vi "校准设置页.vi"() -> ()   [LabVIEW 2016, in "斯坦道氨氮.lvlib"]
uses:
  <vilib>/Analysis/6fits.llb/Curve Fitting Criteria.ctl
  <vilib>/Analysis/NI_AALPro.lvlib
  <vilib>/ptbypt/NI_PtbyPt.lvlib
panel:
  in  "历史数据导入":T1(radio)
  out "校准状态显示":string caption="校准状态"
  out "刷新时间":string
  out "校准状态":T2(ring)
  out "模型刷新":bool
  in  "校准按钮":T1(radio)
  in  "校准导入":bool
  in  "辅助计算":bool
  in  "曲线模型":T3={"标液浓度1"=0.0, "测量吸光度1"=0.0, "样品1启用"=FALSE, "标液浓度2"=0.0, "测量吸光度2"=0.0, "样品2启用"=FALSE, "标液浓度3"=0.0, "测量吸光度3"=0.0, "样品3启用"=FALSE, "标液浓度4"=0.0, "测量吸光度4"=0.0, "样品4启用"=FALSE, "标液浓度5"=0.0, "测量吸光度5"=0.0, "样品5启用"=FALSE, "模型"=enum."线性", "精度"=4.0, "XY图"=[], "拟合公式"="", "r^2"=0.0, "标样一校准时间"=timestamp(0 s since 1904-01-01), "标样二校准时间"=timestamp(0 s since 1904-01-01), "标样三校准时间"=timestamp(0 s since 1904-01-01), "标样四校准时间"=timestamp(0 s since 1904-01-01), "标样五校准时间"=timestamp(0 s since 1904-01-01), "二次方程"={"c"=0.0, "x"=0.0, "x^2"=0.0}, "标定时间"=timestamp(0 s since 1904-01-01)} {"标定时间" format="%<%m/%d/%y %H:%M:%S>T"; "标样五校准时间" format="%<%m/%d/%y %H:%M:%S>T"; "标样四校准时间" format="%<%m/%d/%y %H:%M:%S>T"; "标样三校准时间" format="%<%m/%d/%y %H:%M:%S>T"; "标样二校准时间" format="%<%m/%d/%y %H:%M:%S>T"; "标样一校准时间" format="%<%m/%d/%y %H:%M:%S>T"; "r^2" format="%.7f"; "测量吸光度5" format="%#.6f"; "测量吸光度4" format="%#.6f"; "测量吸光度3" format="%#.6f"; "测量吸光度2" format="%#.6f"; "测量吸光度1" format="%#.6f"}
  in  "测量模式":T4(ring)
  in  "参数下拉列表":u16(ring)
  in  "量程下拉列表":enum16{"低量程", "高量程"}(ring)
  # "校准时间"
  # "标液浓度"
  # "吸光值"
  # "空白"
  # "标样一"
  # "标样二"
  # "零点"
  # "跨度"
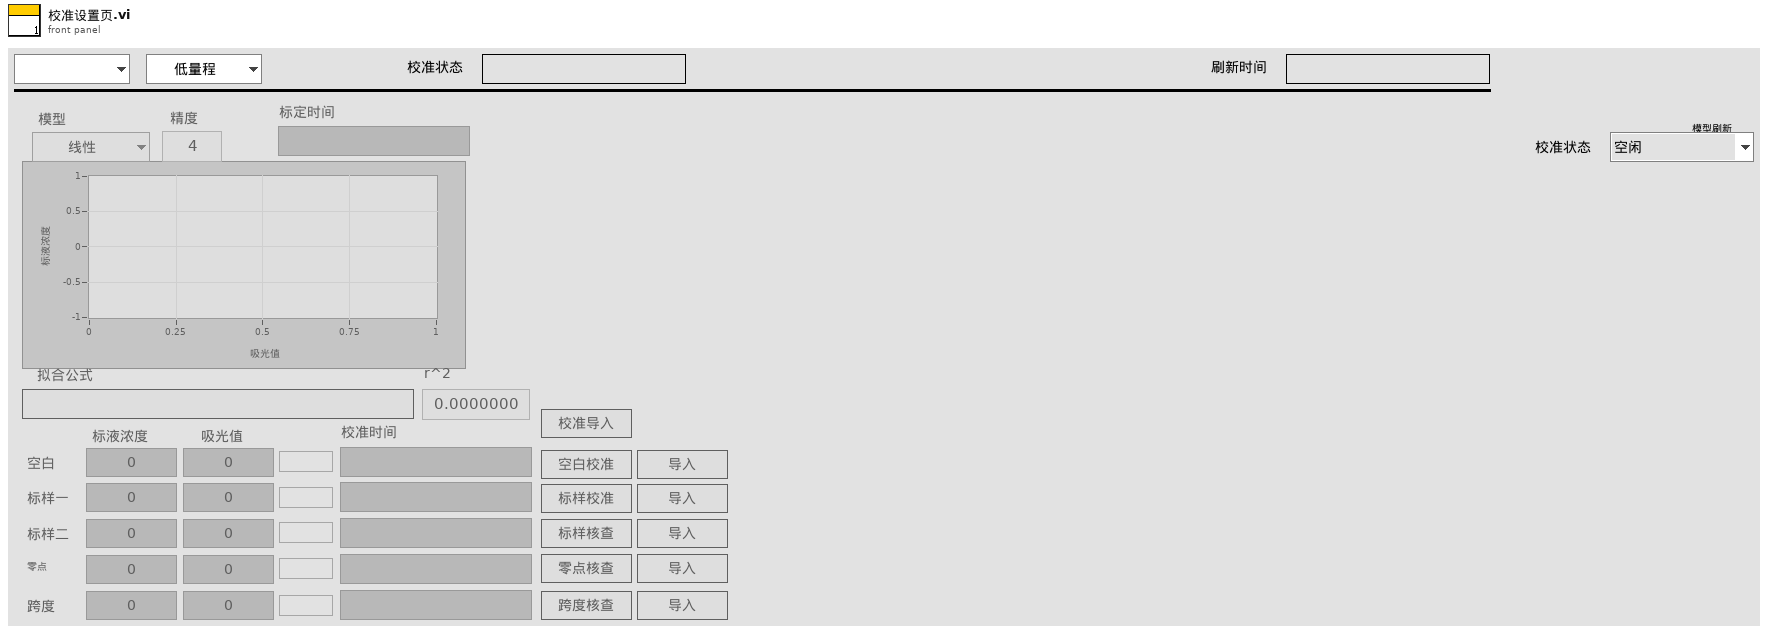
[diagram p1: front panel]
types:
  T1 = enum32{"未选择", "空白校准", "标样校准", "标样核查", "零点核查", "跨度核查"}
  T2 = enum16{"空闲", "初始化", "校准启动", "校准运行中", "测试结束", "获取校准数据", "填充校准数据", "流程结束"}
  T3 = cluster{"标液浓度1":dbl, "测量吸光度1":dbl, "样品1启用":bool, "标液浓度2":dbl, "测量吸光度2":dbl, "样品2启用":bool, "标液浓度3":dbl, "测量吸光度3":dbl, "样品3启用":bool, "标液浓度4":dbl, "测量吸光度4":dbl, "样品4启用":bool, "标液浓度5":dbl, "测量吸光度5":dbl, "样品5启用":bool, "模型":enum32{"线性", "多项式"}, "精度":dbl, "XY图":cluster{"X Values":dbl[], "Y Values":dbl[]}[], "拟合公式":string, "r^2":dbl, "标样一校准时间":timestamp, "标样二校准时间":timestamp, "标样三校准时间":timestamp, "标样四校准时间":timestamp, "标样五校准时间":timestamp, "二次方程":cluster{"c":dbl, "x":dbl, "x^2":dbl}, "标定时间":timestamp}
  T4 = enum16{"跨度核查", "水样测量", "零点核查", "标样核查", "加标回收", "快捷测试", "空白校准", "标样校准"}
  T5 = enum8{"Enabled", "Disabled", "Disabled and Grayed Out"}
  T6 = typedef "LVStringsAndValuesArrayTypeDef_U16.ctl" = cluster{"String":string, "Value":u16}[]
  T7 = cluster{"标液浓度1":dbl, "测量吸光度1":dbl, "样品1启用":bool, "标液浓度2":dbl, "测量吸光度2":dbl, "样品2启用":bool, "标液浓度3":dbl, "测量吸光度3":dbl, "样品3启用":bool, "标液浓度4":dbl, "测量吸光度4":dbl, "样品4启用":bool, "标液浓度5":dbl, "测量吸光度5":dbl, "样品5启用":bool, "模型":enum32{"线性", "多项式"}, "精度":dbl, "XY图":cluster{"X Values":dbl[], "Y Values":dbl[]}[], "拟合公式":string, "r^2":dbl, "标样一校准时间":timestamp, "标样二校准时间":timestamp, "标样三校准时间":timestamp, "标样四校准时间":timestamp, "标样五校准时间":timestamp, "二次方程":cluster{"c":dbl, "x":dbl, "x^2":dbl}, "标定时间":timestamp}[]
  T8 = typedef "NI_AALPro.lvlib/Curve Fitting Criteria.ctl" = u16
  T9 = enum32{"Bad", "Idle", "Run top level", "Running"}
  T10 = cluster{"时间":timestamp, "标液值":dbl, "检测值":dbl, "吸光值":dbl}
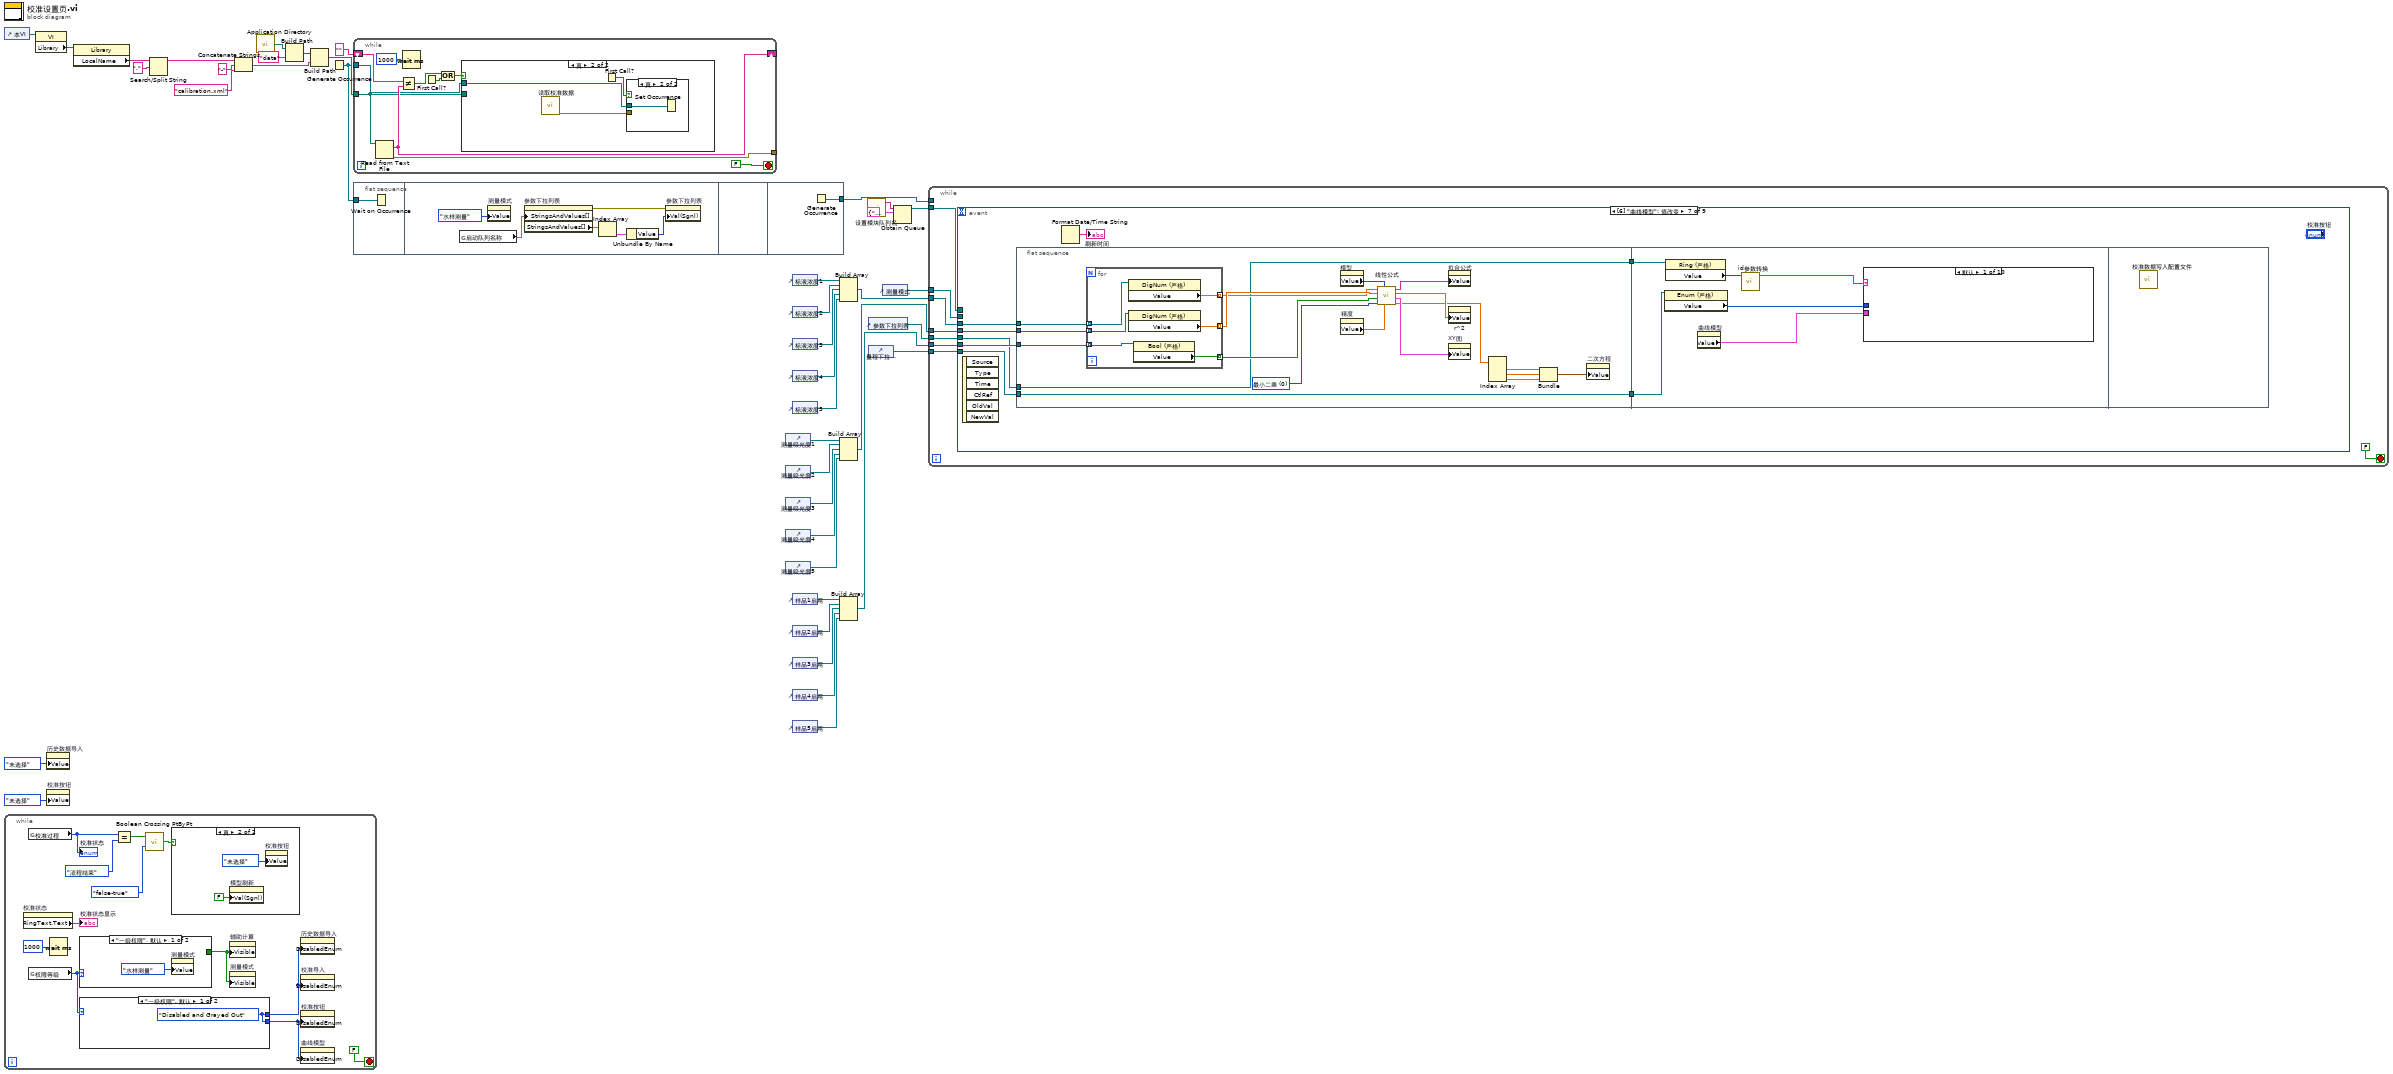
[diagram p0: block diagram]
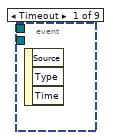
[diagram p4: hidden frame]
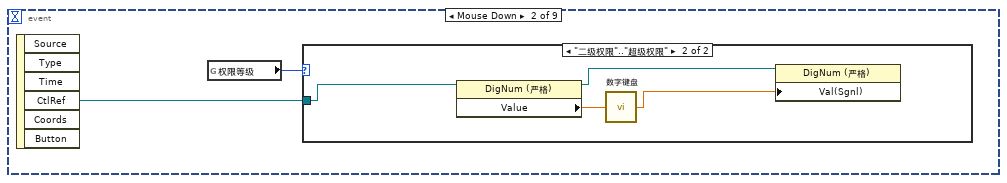
[diagram p5: hidden frame]
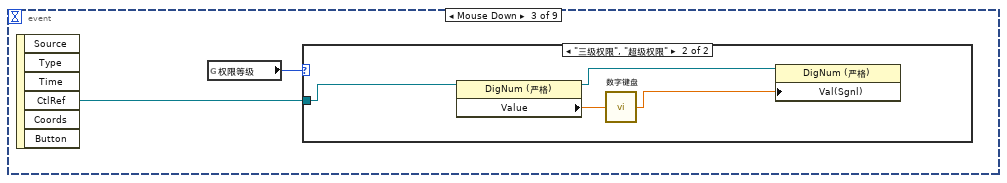
[diagram p7: hidden frame]
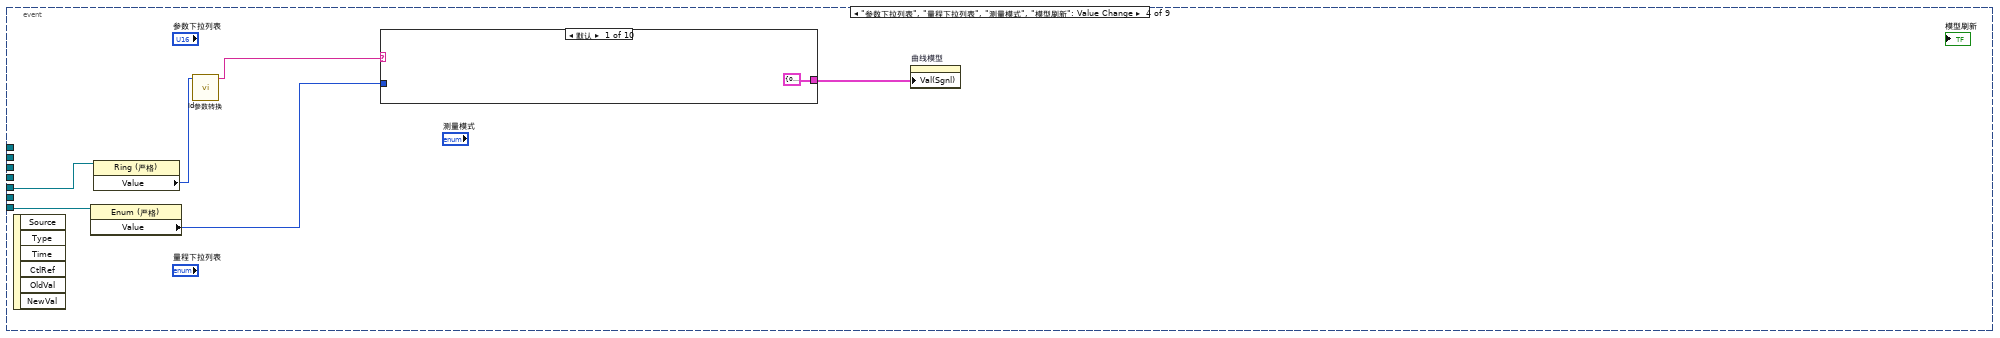
[diagram p9: hidden frame]
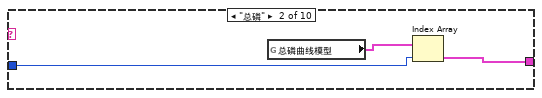
[diagram p10: hidden frame]
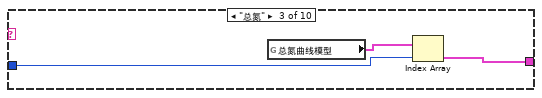
[diagram p11: hidden frame]
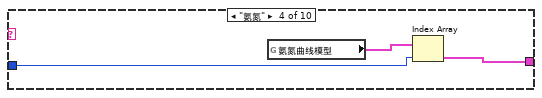
[diagram p12: hidden frame]
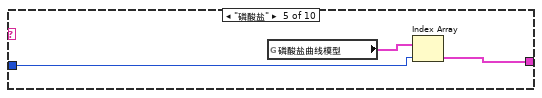
[diagram p13: hidden frame]
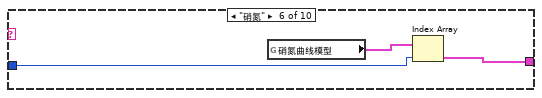
[diagram p14: hidden frame]
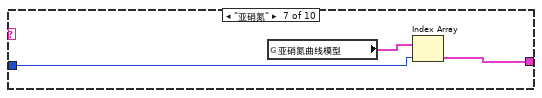
[diagram p15: hidden frame]
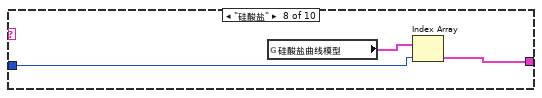
[diagram p16: hidden frame]
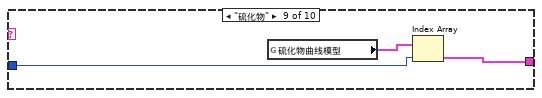
[diagram p17: hidden frame]
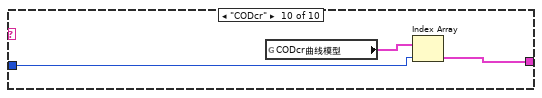
[diagram p18: hidden frame]
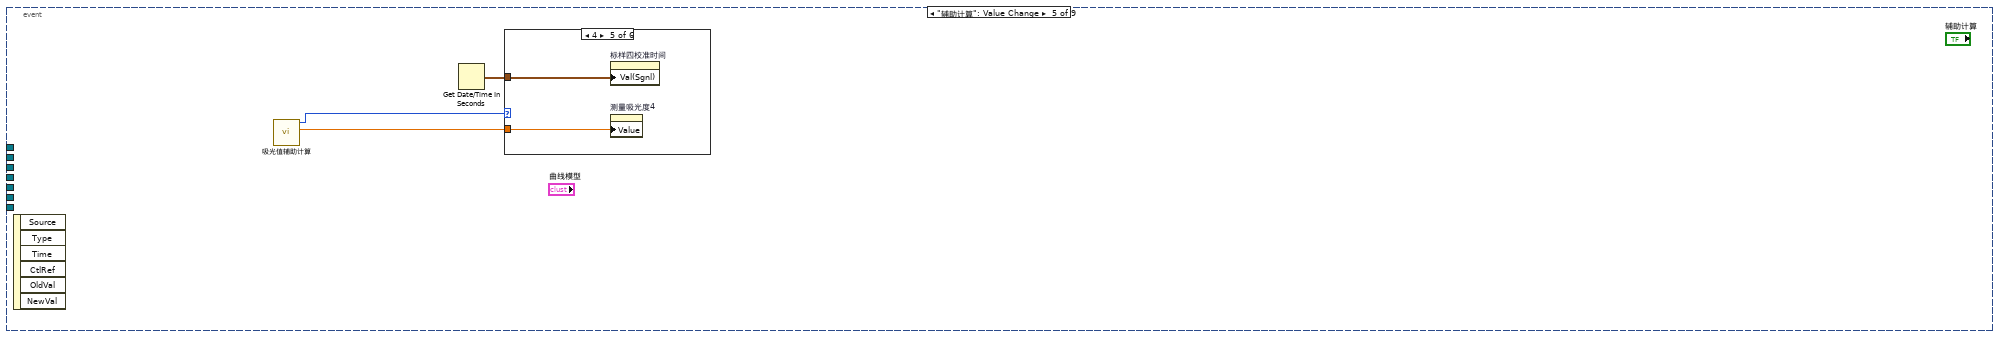
[diagram p19: hidden frame]
diagram:
  n1 = control-ref of="本VI"() -> (w11:refnum<vi>)
  n2 = while {
    stop <- FALSE stop-if-true
    n3 = property on="校准状态" class="Enum (严格)"() -> ("RingText.Text"=→"校准状态显示":string)  [unwired: 2 in, 2 out]
    n4 = global read "VAR总磷总氮全局变量.vi" "校准过程"() -> (w45:T2)
    "校准状态" <- w45
    n5 = global read "VAR总磷总氮全局变量.vi" "权限等级"() -> (w51:enum16{"一级权限", "二级权限", "三级权限", "超级权限"})
    n6 = Wait (ms)(milliseconds to wait=u32 1000 ("等待时间（毫秒）")) -> ()  [unwired: 1 out]
    n7 = case shown="\"一级权限\", 默认" w51 {
      tunnel: [_ TRUE ("可见")] -> w50
      frame "一级权限", Default {
        n8 = property on="测量模式" class="Enum (严格)"("Value"=T4."水样测量" ("测量模式")) -> ()  [unwired: 2 in, 2 out]
      }
      frame "三级权限", "超级权限" {
      }
    }
    n9 = case shown="\"一级权限\", 默认" w51 {
      tunnel: [w58 w59] -> w49
      tunnel: [w58 w59] -> w42
      frame "一级权限", Default {
        w58 = T5."Disabled and Grayed Out" ("禁用")
      }
      frame "二级权限".."超级权限" {
        w59 = T5."Enabled" ("禁用")
      }
    }
    n10 = Equal?(x=w45, y=T2."流程结束" ("校准过程")) -> (x = y?=w48:bool)
    n11 = call <vilib>:"Boolean Crossing PtByPt.vi"("direction"=enum16{"either", "false-true", "true-false"}."false-true", "input"=w48) -> ("crossing"=w46:bool)  [unwired: 1 in]
    n12 = case shown="真" w46 {
      frame False {
      }
      frame True {
        n13 = property on="模型刷新" class="Bool (严格)"("Val(Sgnl)"=FALSE ("值(信号)")) -> ()  [unwired: 2 in, 2 out]
        n14 = property on="校准按钮" class="RadioBtnsControl (严格)"("Value"=T1."未选择" ("校准按钮")) -> ()  [unwired: 2 in, 2 out]
      }
    }
    n15 = property on="辅助计算" class="Bool"("Visible"=w50) -> ()  [unwired: 2 in, 2 out]
    n16 = property on="测量模式" class="Enum (严格)"("Visible"=w50) -> ()  [unwired: 2 in, 2 out]
    n17 = property on="历史数据导入" class="RadioBtnsControl (严格)"("DisabledEnum"=w42) -> ()  [unwired: 2 in, 2 out]
    n18 = property on="校准导入" class="Bool"("DisabledEnum"=w42) -> ()  [unwired: 2 in, 2 out]
    n19 = property on="校准按钮" class="RadioBtnsControl (严格)"("DisabledEnum"=w49) -> ()  [unwired: 2 in, 2 out]
    n20 = property on="曲线模型" class="Clust (严格)"("DisabledEnum"=w49) -> ()  [unwired: 2 in, 2 out]
  }
  n21 = property class="VI"(reference=w11) -> ("Library"=w12:refnum<vi>)  [unwired: 1 in, 2 out]
  n22 = property on="历史数据导入" class="RadioBtnsControl (严格)"("Value"=T1."未选择" ("历史数据导入")) -> ()  [unwired: 2 in, 2 out]
  n23 = property on="校准按钮" class="RadioBtnsControl (严格)"("Value"=T1."未选择" ("校准按钮")) -> ()  [unwired: 2 in, 2 out]
  n24 = property class="Library"(reference=w12) -> ("LocalName"=w9:string)  [unwired: 1 in, 2 out]
  n25 = Search/Split String(string=w9, search string/char (-)="." ("搜索字符串/字符(-)")) -> (substring before match=w7:string)  [unwired: 1 in, 2 out]
  n26 = Concatenate Strings(w7, "-" ("字符串"), "calibration.xml" ("名称或相对路径")) -> (w4:string)
  n27 = call <vilib>:"Application Directory.vi"() -> ("Application Directory"=w13:path)
  n28 = Build Path(base path=w13, name or relative path="data" ("名称或相对路径")) -> (appended path=w10:path)
  n29 = Build Path(base path=w10, name or relative path=w4) -> (appended path=w3:path)
  n30 = Generate Occurrence() -> (w2:refnum<k4>)
  n31 = while {
    shift-right: [w66] -> _
    shift-left: "" -> [w68]
    tunnel: w3 -> [w65]
    tunnel: [w63] -> _
    tunnel: w2 -> [w62]
    stop <- FALSE stop-if-true
    n32 = Read from Text File(file (use dialog)=w65) -> (text=w66:string, error out=w63:errorcluster)  [unwired: 3 in, 2 out]
    n33 = Not Equal?(x=w68, y=w66) -> (x != y?=w67:bool)
    n34 = Wait (ms)(milliseconds to wait=u32 1000 ("等待时间（毫秒）")) -> ()  [unwired: 1 out]
    n35 = First Call?() -> (First Call?: T/F=w60:bool)
    n36 = Or(x=w67, y=w60) -> (x .or. y?=w61:bool)
    n37 = case shown="真" w61 {
      tunnel: w65 -> [_ _]
      tunnel: w62 -> [_ w72]
      frame False {
      }
      frame True {
        n38 = call "读取校准数据.vi"() -> ("错误输出"=w71:errorcluster)  [unwired: 11 in]
        n39 = First Call?() -> (First Call?: T/F=w70:bool)
        n40 = case shown="真" w70 {
          tunnel: w72 -> [_ w73]
          tunnel: w71 -> [_ _]
          frame False {
          }
          frame True {
            n41 = Set Occurrence(w73) -> ()
          }
        }
      }
    }
  }
  n42 = flat-sequence {
    tunnel: w2 -> [w74]
    tunnel: [w81] -> w41
    frame #0 {
      n43 = Wait on Occurrence(2:w74) -> ()  [unwired: 2 in, 1 out]
    }
    frame #1 {
      n44 = global read "总磷总氮断电保存全局变量.vi" "启动队列名称"() -> (w76:cluster{"String":string, "Value":u16}[])
      n45 = property on="测量模式" class="Enum (严格)"("Value"=T4."水样测量" ("测量模式")) -> ()  [unwired: 2 in, 2 out]
      n46 = property on="参数下拉列表" class="Ring (严格)"("StringsAndValues[]"=w76) -> (error out=w79:errorcluster, "StringsAndValues[]"=w77:T6)  [unwired: 2 in, 1 out]
      n47 = Index Array(array=w77) -> (element=w78:cluster{"String":string, "Value":u16})  [unwired: 1 in]
      n48 = Unbundle By Name(w78) -> ("Value"=w80:u16)
      n49 = property on="参数下拉列表" class="Ring (严格)"(error in=w79, "Val(Sgnl)"=w80) -> ()  [unwired: 1 in, 2 out]
    }
    frame #2 {
    }
    frame #3 {
      n50 = Generate Occurrence() -> (w81:refnum<k4>)
    }
  }
  n51 = control-ref of="测量吸光度1"() -> (w30:refnum<vi>)
  n52 = control-ref of="测量吸光度2"() -> (w31:refnum<vi>)
  n53 = control-ref of="测量吸光度3"() -> (w32:refnum<vi>)
  n54 = control-ref of="测量吸光度4"() -> (w33:refnum<vi>)
  n55 = control-ref of="测量吸光度5"() -> (w34:refnum<vi>)
  n56 = control-ref of="标液浓度1"() -> (w28:refnum<vi>)
  n57 = control-ref of="标液浓度2"() -> (w27:refnum<vi>)
  n58 = control-ref of="标液浓度3"() -> (w26:refnum<vi>)
  n59 = control-ref of="标液浓度4"() -> (w25:refnum<vi>)
  n60 = control-ref of="标液浓度5"() -> (w24:refnum<vi>)
  n61 = control-ref of="样品1启用"() -> (w40:refnum<vi>)
  n62 = control-ref of="样品2启用"() -> (w39:refnum<vi>)
  n63 = control-ref of="样品3启用"() -> (w38:refnum<vi>)
  n64 = control-ref of="样品4启用"() -> (w37:refnum<vi>)
  n65 = control-ref of="样品5启用"() -> (w36:refnum<vi>)
  n66 = Build Array(w28, w27, w26, w25, w24) -> (w23:refnum<vi>[])
  n67 = Build Array(w30, w31, w32, w33, w34) -> (w29:refnum<vi>[])
  n68 = Build Array(w40, w39, w38, w37, w36) -> (w35:refnum<vi>[])
  n69 = call "设置模块队列名.vi"() -> ("Msg"=w21:string)  [unwired: 5 in]
  n70 = control-ref of="参数下拉列表"() -> (w18:refnum<vi>)
  n71 = control-ref of="量程下拉列表"() -> (w16:refnum<vi>)
  n72 = control-ref of="测量模式"() -> (w17:refnum<vi>)
  n73 = Obtain Queue(name (unnamed)=w21, element data type=cluster{"命令":string, "data":variant} {"命令"="", "data"=variant}) -> (queue out=w20:refnum<queue>)  [unwired: 3 in, 2 out]
  n74 = while {
    tunnel: w41 -> [_]
    tunnel: w18 -> [w88]
    tunnel: w35 -> [w87]
    tunnel: w29 -> [w86]
    tunnel: w23 -> [w85]
    tunnel: w17 -> [w84]
    tunnel: w16 -> [w83]
    tunnel: w20 -> [w82]
    stop <- FALSE stop-if-true
    n75 = event shown="[6] \"曲线模型\": 值改变" {
      selector: _ -> [_ _ _ _ _ _ _ _ _]
      dyn-events: _ -> [_ _ _ _ _ _ _ _ _]
      timeout: _ -> [_ _ _ _ _ _ _ _ _]
      tunnel: w88 -> [_ _ _ w106 _ w161 w206 w283 w321]
      tunnel: w87 -> [_ _ _ _ _ _ w210 _ _]
      tunnel: w86 -> [_ _ _ _ _ _ w209 _ _]
      tunnel: w85 -> [_ _ _ _ _ _ w208 _ _]
      tunnel: w84 -> [_ _ _ _ _ w159 _ w278 w316]
      tunnel: w83 -> [_ _ _ w104 _ w157 w204 w282 w320]
      tunnel: w82 -> [_ _ _ _ _ _ _ w284 w322]
      event Timeout {
        n76 = event-data() -> ()  [unwired: 1 in, 3 out]
      }
      event "曲线模型.标液浓度1", "曲线模型.标液浓度2", "曲线模型.标液浓度3", "曲线模型.标液浓度4", "曲线模型.标液浓度5", "曲线模型.精度": Mouse Down {
        n77 = event-data() -> ("CtlRef"=w91:refnum<vi>)  [unwired: 1 in, 5 out]
        n78 = global read "VAR总磷总氮全局变量.vi" "权限等级"() -> (w90:enum16{"一级权限", "二级权限", "三级权限", "超级权限"})
        n79 = case shown="\"二级权限\"..\"超级权限\"" w90 {
          tunnel: w91 -> [_ w95]
          frame "一级权限", Default {
          }
          frame "二级权限".."超级权限" {
            n80 = property class="DigNum (严格)"(reference=w95) -> (reference out=w93:refnum<vi>, "Value"=w94:dbl)  [unwired: 1 in, 1 out]
            n81 = call "数字键盘.vi"("OldNumber"=w94) -> ("NewNumber"=w92:dbl)
            n82 = property class="DigNum (严格)"(reference=w93, "Val(Sgnl)"=w92) -> ()  [unwired: 1 in, 2 out]
          }
        }
      }
      event "曲线模型.测量吸光度1", "曲线模型.测量吸光度2", "曲线模型.测量吸光度3", "曲线模型.测量吸光度4", "曲线模型.测量吸光度5": Mouse Down {
        n83 = event-data() -> ("CtlRef"=w97:refnum<vi>)  [unwired: 1 in, 5 out]
        n84 = global read "VAR总磷总氮全局变量.vi" "权限等级"() -> (w96:enum16{"一级权限", "二级权限", "三级权限", "超级权限"})
        n85 = case shown="\"三级权限\", \"超级权限\"" w96 {
          tunnel: w97 -> [_ w101]
          frame "一级权限", Default {
          }
          frame "三级权限", "超级权限" {
            n86 = property class="DigNum (严格)"(reference=w101) -> (reference out=w99:refnum<vi>, "Value"=w100:dbl)  [unwired: 1 in, 1 out]
            n87 = call "数字键盘.vi"("OldNumber"=w100) -> ("NewNumber"=w98:dbl)
            n88 = property class="DigNum (严格)"(reference=w99, "Val(Sgnl)"=w98) -> ()  [unwired: 1 in, 2 out]
          }
        }
      }
      event "参数下拉列表", "量程下拉列表", "测量模式", "模型刷新": Value Change {
        n89 = event-data() -> ()  [unwired: 1 in, 6 out]
        n90 = property class="Enum (严格)"(reference=w104) -> ("Value"=w102:enum16{"低量程", "高量程"})  [unwired: 1 in, 2 out]
        n91 = property class="Ring (严格)"(reference=w106) -> ("Value"=w107:u16)  [unwired: 1 in, 2 out]
        n92 = call "id参数转换.vi"("id"=w107) -> ("table输出"=w105:string)  [unwired: 9 in, 1 out]
        n93 = case shown="默认" w105 {
          tunnel: w102 -> [_ w109 w112 w115 w118 w121 w124 w127 w130 w133]
          tunnel: [T3 {"标液浓度1"=0.0, "测量吸光度1"=0.0, "样品1启用"=FALSE, "标液浓度2"=0.0, "测量吸光度2"=0.0, "样品2启用"=FALSE, "标液浓度3"=0.0, "测量吸光度3"=0.0, "样品3启用"=FALSE, "标液浓度4"=0.0, "测量吸光度4"=0.0, "样品4启用"=FALSE, "标液浓度5"=0.0, "测量吸光度5"=0.0, "样品5启用"=FALSE, "模型"=enum."线性", "精度"=0.0, "XY图"=[], "拟合公式"="", "r^2"=0.0, "标样一校准时间"=timestamp(0 s since 1904-01-01), "标样二校准时间"=timestamp(0 s since 1904-01-01), "标样三校准时间"=timestamp(0 s since 1904-01-01), "标样四校准时间"=timestamp(0 s since 1904-01-01), "标样五校准时间"=timestamp(0 s since 1904-01-01), "二次方程"={"c"=0.0, "x"=0.0, "x^2"=0.0}, "标定时间"=timestamp(0 s since 1904-01-01)} ("总磷曲线模型") w110 w113 w116 w119 w122 w125 w128 w131 w134] -> w103
          frame Default {
          }
          frame "总磷" {
            n94 = global read "校准数据全局变量.vi" "总磷曲线模型"() -> (w111:T7)
            n95 = Index Array(array=w111, index=w109) -> (element=w110:T3)
          }
          frame "总氮" {
            n96 = global read "校准数据全局变量.vi" "总氮曲线模型"() -> (w114:T7)
            n97 = Index Array(array=w114, index=w112) -> (element=w113:T3)
          }
          frame "氨氮" {
            n98 = global read "校准数据全局变量.vi" "氨氮曲线模型"() -> (w117:T7)
            n99 = Index Array(array=w117, index=w115) -> (element=w116:T3)
          }
          frame "磷酸盐" {
            n100 = global read "校准数据全局变量.vi" "磷酸盐曲线模型"() -> (w120:T7)
            n101 = Index Array(array=w120, index=w118) -> (element=w119:T3)
          }
          frame "硝氮" {
            n102 = global read "校准数据全局变量.vi" "硝氮曲线模型"() -> (w123:T7)
            n103 = Index Array(array=w123, index=w121) -> (element=w122:T3)
          }
          frame "亚硝氮" {
            n104 = global read "校准数据全局变量.vi" "亚硝氮曲线模型"() -> (w126:T7)
            n105 = Index Array(array=w126, index=w124) -> (element=w125:T3)
          }
          frame "硅酸盐" {
            n106 = global read "校准数据全局变量.vi" "硅酸盐曲线模型"() -> (w129:T7)
            n107 = Index Array(array=w129, index=w127) -> (element=w128:T3)
          }
          frame "硫化物" {
            n108 = global read "校准数据全局变量.vi" "硫化物曲线模型"() -> (w132:T7)
            n109 = Index Array(array=w132, index=w130) -> (element=w131:T3)
          }
          frame "CODcr" {
            n110 = global read "校准数据全局变量.vi" "CODcr曲线模型"() -> (w135:T7)
            n111 = Index Array(array=w135, index=w133) -> (element=w134:T3)
          }
        }
        n112 = property on="曲线模型" class="Clust (严格)"("Val(Sgnl)"=w103) -> ()  [unwired: 2 in, 2 out]
      }
      event "辅助计算": Value Change {
        n113 = event-data() -> ()  [unwired: 1 in, 6 out]
        n114 = call "吸光值辅助计算.vi"() -> ("X"=w137:dbl, "吸光值导出"=w138:u16)  [unwired: 10 in]
        n115 = Get Date/Time In Seconds() -> (seconds since 1Jan1904=w136:timestamp)
        n116 = case shown="4" w138 {
          tunnel: w137 -> [_ w140 w142 w144 w146 w148]
          tunnel: w136 -> [_ w139 w141 w143 w145 w147]
          frame 0, Default {
          }
          frame 1 {
            n117 = property on="标样一校准时间" class="AbsTime (严格)"("Val(Sgnl)"=w139) -> ()  [unwired: 2 in, 2 out]
            n118 = property on="测量吸光度1" class="DigNum (严格)"("Value"=w140) -> ()  [unwired: 2 in, 2 out]
          }
          frame 2 {
            n119 = property on="标样二校准时间" class="AbsTime (严格)"("Val(Sgnl)"=w141) -> ()  [unwired: 2 in, 2 out]
            n120 = property on="测量吸光度2" class="DigNum (严格)"("Value"=w142) -> ()  [unwired: 2 in, 2 out]
          }
          frame 3 {
            n121 = property on="标样三校准时间" class="AbsTime (严格)"("Val(Sgnl)"=w143) -> ()  [unwired: 2 in, 2 out]
            n122 = property on="测量吸光度3" class="DigNum (严格)"("Value"=w144) -> ()  [unwired: 2 in, 2 out]
          }
          frame 4 {
            n123 = property on="标样四校准时间" class="AbsTime (严格)"("Val(Sgnl)"=w145) -> ()  [unwired: 2 in, 2 out]
            n124 = property on="测量吸光度4" class="DigNum (严格)"("Value"=w146) -> ()  [unwired: 2 in, 2 out]
          }
          frame 5 {
            n125 = property on="标样五校准时间" class="AbsTime (严格)"("Val(Sgnl)"=w147) -> ()  [unwired: 2 in, 2 out]
            n126 = property on="测量吸光度5" class="DigNum (严格)"("Value"=w148) -> ()  [unwired: 2 in, 2 out]
          }
        }
      }
      event "校准导入": Value Change {
        n127 = event-data() -> ()  [unwired: 1 in, 6 out]
        n128 = property class="Enum (严格)"(reference=w159) -> ("Value"=w158:T4)  [unwired: 1 in, 2 out]
        n129 = property class="Enum (严格)"(reference=w157) -> ("Value"=w156:enum16{"低量程", "高量程"})  [unwired: 1 in, 2 out]
        n130 = property class="Ring (严格)"(reference=w161) -> ("Value"=w160:u16)  [unwired: 1 in, 2 out]
        n131 = property on="二次方程" class="Clust (严格)"() -> ("Value"=w150:cluster{"c":dbl, "x":dbl, "x^2":dbl})  [unwired: 2 in, 2 out]
        n132 = Unbundle By Name(w150) -> ("x^2"=w152:dbl, "x"=w153:dbl, "c"=w154:dbl)
        n133 = Bundle By Name(cluster=cluster{"X^2":dbl, "X":dbl, "b":dbl} {"X^2"=0.0, "X"=0.0, "b"=0.0} ("公式"), "X^2"=w152, "X"=w153, "b"=w154) -> (w149:cluster{"X^2":dbl, "X":dbl, "b":dbl})
        n134 = global read "VAR总磷总氮全局变量.vi" "权限等级"() -> (w155:enum16{"一级权限", "二级权限", "三级权限", "超级权限"})
        n135 = case shown="\"三级权限\", \"超级权限\"" w155 {
          tunnel: w160 -> [w170 w202]
          tunnel: w158 -> [w169 w201]
          tunnel: w156 -> [w168 w200]
          tunnel: w149 -> [w162 w199]
          frame "一级权限", Default {
            n136 = Cluster To Array(cluster=w162) -> (array=w167:dbl[])
            n137 = Add Array Elements(numeric array=w167) -> (sum=w166:dbl)
            n138 = Equal To 0?(x=w166) -> (x = 0?=w164:bool)
            n139 = Not A Number/Path/Refnum?(number/path/refnum=w166) -> (NaN/Path/Refnum?=w165:bool)
            n140 = Or(x=w164, y=w165) -> (x .or. y?=w163:bool)
            n141 = case shown="假" w163 {
              tunnel: w170 -> [w176 _]
              tunnel: w169 -> [w175 _]
              tunnel: w168 -> [w174 _]
              tunnel: w162 -> [w171 _]
              frame False {
                n142 = Two Button Dialog(message="请再一次确认是否导入" ("消息")) -> (T button?=w172:bool)  [unwired: 2 in]
                n143 = case shown="真" w172 {
                  tunnel: w176 -> [_ w178]
                  tunnel: w175 -> [_ w184]
                  tunnel: w174 -> [_ w177]
                  tunnel: w171 -> [_ w179]
                  frame False {
                  }
                  frame True {
                    n144 = for {
                      N: 8 -> [_]
                      tunnel: w178 -> [w190]
                      tunnel: w184 -> [_]
                      tunnel: w177 -> [w189]
                      shift-right: [w188] -> w182
                      shift-left: errorcluster {"status"=FALSE, "code"=0, "source"=""} ("error out") -> [w185]
                      tunnel: w179 -> [w186]
                      i -> [w187]
                      n145 = call "总磷总氮公式写入.vi"("公式"=w186, "error in (no error)"=w185, "量程"=w189, "测量模式"=w187, "测量参数"=w190) -> ("error out"=w188:errorcluster)  [unwired: 6 in]
                    }
                    n146 = case shown="无错误" w182 {
                      tunnel: ["写入成功" "写入失败"] -> w183
                      tunnel: w178 -> [w194 _]
                      tunnel: w177 -> [w193 _]
                      frame No Error {
                        n147 = Get Date/Time In Seconds() -> (seconds since 1Jan1904=w195:timestamp)
                        n148 = property on="标定时间" class="AbsTime (严格)"("Val(Sgnl)"=w195) -> (error out=w191:errorcluster)  [unwired: 2 in, 1 out]
                        n149 = property on="曲线模型" class="Clust (严格)"(error in=w191) -> ("Value"=w192:T3)  [unwired: 1 in, 2 out]
                        n150 = call "校准记录.vi"("曲线模型"=w192, "量程"=w193, "校准参数"=w194) -> ()  [unwired: 8 in, 1 out]
                      }
                      frame Error {
                      }
                    }
                    n151 = One Button Dialog(message=w183) -> ()  [unwired: 1 in, 1 out]
                  }
                }
              }
              frame True {
                n152 = One Button Dialog(message="校准数据异常，请重新校准！" ("消息")) -> ()  [unwired: 1 in, 1 out]
              }
            }
          }
          frame "三级权限", "超级权限" {
            n153 = call "公式复合写入.vi"("公式"=w199, "量程下拉列表"=w200, "测量模式"=w201, "参数下拉列表"=w202) -> ()  [unwired: 8 in]
          }
        }
      }
      event "曲线模型": Value Change {
        n154 = event-data() -> ()  [unwired: 1 in, 6 out]
        n155 = flat-sequence {
          tunnel: w210 -> [w229]
          tunnel: w209 -> [w227]
          tunnel: w208 -> [w225]
          tunnel: [w212] -> w207
          tunnel: w206 -> [w212]
          tunnel: [w211] -> w205
          tunnel: w204 -> [w211]
          tunnel: w207 -> [w241]
          tunnel: w205 -> [w238]
          frame #0 {
            w221 = T8 0 items=["最小二乘", "最小绝对残差", "Bisquare"] ("method")
            n156 = for {
              tunnel: w229 -> [w235] mode=indexing
              tunnel: [w234] -> w228 mode=indexing
              tunnel: w227 -> [w233] mode=indexing
              tunnel: [w232] -> w226 mode=indexing
              tunnel: w225 -> [w231] mode=indexing
              tunnel: [w230] -> w224 mode=indexing
              n157 = property class="DigNum (严格)"(reference=w231) -> ("Value"=w230:dbl)  [unwired: 1 in, 2 out]
              n158 = property class="DigNum (严格)"(reference=w233) -> ("Value"=w232:dbl)  [unwired: 1 in, 2 out]
              n159 = property class="Bool (严格)"(reference=w235) -> ("Value"=w234:bool)  [unwired: 1 in, 2 out]
            }
            n160 = property on="模型" class="Enum (严格)"() -> ("Value"=w223:enum32{"线性", "多项式"})  [unwired: 2 in, 2 out]
            n161 = property on="精度" class="DigNum (严格)"() -> ("Value"=w222:dbl)  [unwired: 2 in, 2 out]
            n162 = call "线性公式.vi"("精度"=w222, "模型"=w223, "method"=w221, "启用"=w228, "监测浓度"=w226, "标液浓度"=w224) -> ("Polynomial Coefficients 2"=w217:dbl[], "XY图"=w218:cluster{"X Values":dbl[], "Y Values":dbl[]}[], "r^2"=w219:dbl, "拟合方程"=w220:string)  [unwired: 2 in]
            n163 = property on="拟合公式" class="Str"("Value"=w220) -> ()  [unwired: 2 in, 2 out]
            n164 = property on="r^2" class="DigNum (严格)"("Value"=w219) -> ()  [unwired: 2 in, 2 out]
            n165 = property on="XY图" class="XYGraph (严格)"("Value"=w218) -> ()  [unwired: 2 in, 2 out]
            n166 = Index Array(array=w217) -> (element #1=w216:dbl, element #2=w215:dbl, element #3=w214:dbl)  [unwired: 3 in]
            n167 = Bundle("slope"=w216, "slope"=w215, "slope"=w214) -> (w213:cluster{"slope":dbl, "slope":dbl, "slope":dbl})  [unwired: 1 in]
            n168 = property on="二次方程" class="Clust (严格)"("Value"=w213) -> ()  [unwired: 2 in, 2 out]
          }
          frame #1 {
            n169 = property class="Enum (严格)"(reference=w238) -> ("Value"=w237:enum16{"低量程", "高量程"})  [unwired: 1 in, 2 out]
            n170 = property class="Ring (严格)"(reference=w241) -> ("Value"=w240:u16)  [unwired: 1 in, 2 out]
            n171 = property on="曲线模型" class="Clust (严格)"() -> ("Value"=w236:T3)  [unwired: 2 in, 2 out]
            n172 = call "id参数转换.vi"("id"=w240) -> ("table输出"=w239:string)  [unwired: 9 in, 1 out]
            n173 = case shown="默认" w239 {
              tunnel: w236 -> [_ w243 w249 w252 w255 w259 w263 w267 w271 w276]
              tunnel: w237 -> [_ w242 w246 w250 w254 w258 w262 w266 w270 w274]
              frame Default {
              }
              frame "总磷" {
                n174 = global read "校准数据全局变量.vi" "总磷曲线模型"() -> (w244:T7)
                n175 = Replace Array Subset(array=w244, new element=w243, index=w242) -> (w245:T7)
                n176 = global write "校准数据全局变量.vi" "总磷曲线模型"(w245) -> ()
              }
              frame "总氮" {
                n177 = global read "校准数据全局变量.vi" "总氮曲线模型"() -> (w248:T7)
                n178 = Replace Array Subset(array=w248, new element=w249, index=w246) -> (w247:T7)
                n179 = global write "校准数据全局变量.vi" "总氮曲线模型"(w247) -> ()
              }
              frame "氨氮" {
                n180 = global read "校准数据全局变量.vi" "氨氮曲线模型"() -> (w253:T7)
                n181 = Replace Array Subset(array=w253, new element=w252, index=w250) -> (w251:T7)
                n182 = global write "校准数据全局变量.vi" "氨氮曲线模型"(w251) -> ()
              }
              frame "磷酸盐" {
                n183 = global read "校准数据全局变量.vi" "磷酸盐曲线模型"() -> (w257:T7)
                n184 = Replace Array Subset(array=w257, new element=w255, index=w254) -> (w256:T7)
                n185 = global write "校准数据全局变量.vi" "磷酸盐曲线模型"(w256) -> ()
              }
              frame "硝氮" {
                n186 = global read "校准数据全局变量.vi" "硝氮曲线模型"() -> (w261:T7)
                n187 = Replace Array Subset(array=w261, new element=w259, index=w258) -> (w260:T7)
                n188 = global write "校准数据全局变量.vi" "硝氮曲线模型"(w260) -> ()
              }
              frame "亚硝氮" {
                n189 = global read "校准数据全局变量.vi" "亚硝氮曲线模型"() -> (w265:T7)
                n190 = Replace Array Subset(array=w265, new element=w263, index=w262) -> (w264:T7)
                n191 = global write "校准数据全局变量.vi" "亚硝氮曲线模型"(w264) -> ()
              }
              frame "硅酸盐" {
                n192 = global read "校准数据全局变量.vi" "硅酸盐曲线模型"() -> (w269:T7)
                n193 = Replace Array Subset(array=w269, new element=w267, index=w266) -> (w268:T7)
                n194 = global write "校准数据全局变量.vi" "硅酸盐曲线模型"(w268) -> ()
              }
              frame "硫化物" {
                n195 = global read "校准数据全局变量.vi" "硫化物曲线模型"() -> (w273:T7)
                n196 = Replace Array Subset(array=w273, new element=w271, index=w270) -> (w272:T7)
                n197 = global write "校准数据全局变量.vi" "硫化物曲线模型"(w272) -> ()
              }
              frame "CODcr" {
                n198 = global read "校准数据全局变量.vi" "CODcr曲线模型"() -> (w277:T7)
                n199 = Replace Array Subset(array=w277, new element=w276, index=w274) -> (w275:T7)
                n200 = global write "校准数据全局变量.vi" "CODcr曲线模型"(w275) -> ()
              }
            }
          }
          frame #2 {
            n201 = call "校准数据写入配置文件.vi"() -> ()  [unwired: 11 in, 1 out]
          }
        }
        n202 = Format Date/Time String() -> (date/time string=→"刷新时间":string)  [unwired: 3 in]
      }
      event "校准按钮": Value Change {
        n203 = event-data() -> ("NewVal"=w279:T1)  [unwired: 1 in, 5 out]
        n204 = Not Equal?(x=w279, y=T1."未选择") -> (x != y?=w280:bool)
        n205 = case shown="真" w280 {
          tunnel: w284 -> [_ _]
          tunnel: w283 -> [_ w291]
          tunnel: w282 -> [_ w290]
          tunnel: w279 -> [_ w288]
          tunnel: w278 -> [_ w289]
          frame False {
          }
          frame True {
            n206 = property on="校准按钮" class="RadioBtnsControl (严格)"("Value"=T1."未选择" ("校准按钮")) -> ()  [unwired: 2 in, 2 out]
            n207 = Two Button Dialog(message="按确认立刻启动校准" ("消息")) -> (T button?=w286:bool)  [unwired: 2 in]
            n208 = case shown="真" w286 {
              tunnel: w291 -> [_ w302]
              tunnel: w290 -> [_ w301]
              tunnel: w289 -> [_ w300]
              tunnel: w288 -> [_ w296]
              frame False {
              }
              frame True {
                n209 = property class="Enum (严格)"(reference=w300) -> ("Value"=w294:T4)  [unwired: 1 in, 2 out]
                n210 = property class="Enum (严格)"(reference=w301) -> ("Value"=w293:enum16{"低量程", "高量程"})  [unwired: 1 in, 2 out]
                n211 = property class="Ring (严格)"(reference=w302) -> ("Value"=w295:u16)  [unwired: 1 in, 2 out]
                n212 = vi-ref "校准流程.vi"() -> (w297:refnum<vi>)
                n213 = local read "曲线模型"() -> (w292:T3)
                n214 = property class="VI"(reference=w297) -> ("Name"=w298:string, "Exec.State"=w299:T9)  [unwired: 1 in, 2 out]
                n215 = case shown="\"Bad\", 默认" w299 {
                  tunnel: w298 -> [_ w315]
                  tunnel: w296 -> [_ w308]
                  tunnel: w295 -> [_ w307]
                  tunnel: w294 -> [_ w306]
                  tunnel: w293 -> [_ w305]
                  tunnel: w292 -> [_ w304]
                  frame "Bad", Default {
                    n216 = One Button Dialog(message="正在校准，请在校准完成后操作！" ("消息")) -> ()  [unwired: 1 in, 1 out]
                  }
                  frame "Idle" {
                    n217 = Open VI Reference(type specifier VI Refnum (for type only)=refnum<vi> refnum, vi path=w315, options=128 ("选项")) -> (vi reference=w313:refnum<vi>, error out=w312:errorcluster)  [unwired: 3 in]
                    n218 = call-by-ref "开始异步调用"(reference=w313, error in=w312, "校准模式"=w308, "参数下拉列表"=w307, "测量模式"=w306, "量程下拉列表"=w305, "曲线模型"=w304) -> (reference out=w310:refnum<vi>, error out=w311:errorcluster)  [unwired: 11 in]
                    n219 = Close Reference(reference=w310, error in (no error)=w311) -> ()  [unwired: 1 out]
                  }
                }
              }
            }
          }
        }
      }
      event "历史数据导入": Value Change {
        n220 = event-data() -> ("NewVal"=w317:T1)  [unwired: 1 in, 5 out]
        n221 = Not Equal?(x=w317, y=T1."未选择") -> (x != y?=w318:bool)
        n222 = case shown="真" w318 {
          tunnel: w322 -> [_ _]
          tunnel: w321 -> [_ w330]
          tunnel: w320 -> [_ _]
          tunnel: w317 -> [_ w329]
          tunnel: w316 -> [_ _]
          frame False {
          }
          frame True {
            n223 = property class="Ring (严格)"(reference=w330) -> ("Value"=w328:u16)  [unwired: 1 in, 2 out]
            n224 = case shown="\"跨度核查\"" w329 {
              tunnel: [T4."水样测量" ("测量模式") T4."空白校准" ("测量模式") T4."标样校准" ("测量模式") T4."标样核查" ("测量模式") T4."零点核查" ("测量模式") T4."跨度核查" ("测量模式")] -> w326
              frame "未选择", Default {
              }
              frame "空白校准" {
              }
              frame "标样校准" {
              }
              frame "标样核查" {
              }
              frame "零点核查" {
              }
              frame "跨度核查" {
              }
            }
            n225 = property on="历史数据导入" class="RadioBtnsControl (严格)"("Value"=T1."未选择" ("历史数据导入")) -> ()  [unwired: 2 in, 2 out]
            n226 = call "id参数转换.vi"("id"=w328) -> ("table输出"=w327:string)  [unwired: 9 in, 1 out]
            n227 = call "校准数据选择表.vi"("测量模式"=w326, "table"=w327) -> ("布尔"=w325:bool, "输出"=w324:T10)  [unwired: 8 in]
            n228 = case shown="真" w325 {
              tunnel: w324 -> [_ w334]
              tunnel: w329 -> [_ w337]
              frame False {
              }
              frame True {
                n229 = Unbundle By Name(w334) -> ("时间"=w333:timestamp, "标液值"=w332:dbl, "吸光值"=w331:dbl)
                n230 = property on="曲线模型" class="Clust (严格)"() -> ("Value"=w335:T3)  [unwired: 2 in, 2 out]
                n231 = case shown="\"标样核查\"" w337 {
                  tunnel: [w338 w342 w347 w352 w357 w362] -> w336
                  tunnel: w335 -> [w338 w343 w348 w353 w358 w363]
                  tunnel: w333 -> [_ w341 w346 w351 w356 w361]
                  tunnel: w332 -> [_ w340 w345 w350 w355 w360]
                  tunnel: w331 -> [_ w339 w344 w349 w354 w359]
                  frame "未选择", Default {
                  }
                  frame "空白校准" {
                    n232 = Bundle By Name(cluster=w343, "标样一校准时间"=w341, "标液浓度1"=w340, "测量吸光度1"=w339) -> (w342:T3)
                  }
                  frame "标样校准" {
                    n233 = Bundle By Name(cluster=w348, "标样二校准时间"=w346, "标液浓度2"=w345, "测量吸光度2"=w344) -> (w347:T3)
                  }
                  frame "标样核查" {
                    n234 = Bundle By Name(cluster=w353, "标样三校准时间"=w351, "标液浓度3"=w350, "测量吸光度3"=w349) -> (w352:T3)
                  }
                  frame "零点核查" {
                    n235 = Bundle By Name(cluster=w358, "标样四校准时间"=w356, "标液浓度4"=w355, "测量吸光度4"=w354) -> (w357:T3)
                  }
                  frame "跨度核查" {
                    n236 = Bundle By Name(cluster=w363, "标样五校准时间"=w361, "标液浓度5"=w360, "测量吸光度5"=w359) -> (w362:T3)
                  }
                }
                n237 = property on="曲线模型" class="Clust (严格)"("Val(Sgnl)"=w336) -> ()  [unwired: 2 in, 2 out]
              }
            }
          }
        }
      }
    }
  }
